vi "Panel Controller.vi"(5 "Show Event":refnum<user-event>, 7 "Stop Event":refnum<user-event>, 10 "Panel":refnum<class "Panel.lvclass">) -> ()   [LabVIEW 2017, in "1. Basic Panels.lvlib"]
doc: "This is a basic panel. \n\nIt doesn't know what type of panel it is until runtime, this means that whoever launches this VI can define what type of panel it will be.\n----\nCopyright: MGI 2016\nAuthor: Derek Trepanier"
uses:
  1. Basic Panels.lvlib
  panel-manager/Source/Panel/Panel.lvclass
  panel-manager/Source/Panel Helper/Panel Helper.lvclass
  panel-manager/Source/Deferer/Deferer.lvclass
  panel-manager/Source/Cursor/Cursor.lvclass
panel:
  out "Numeric":i32
  in  "Mouse Busy for 1000ms":bool
  in  "Mouse Busy for 500ms":bool
  in  "Defer for 1000ms":bool
  in  "Defer for 500ms":bool
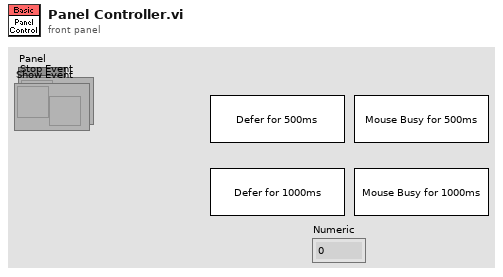
[diagram p1: front panel]
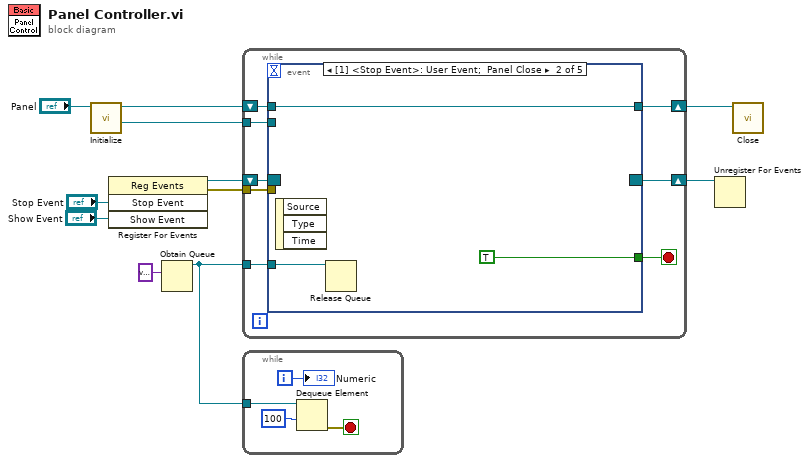
[diagram p0: block diagram]
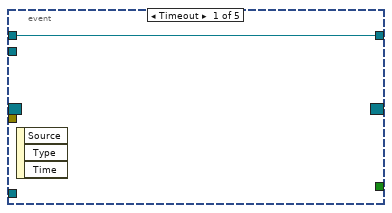
[diagram p2: hidden frame]
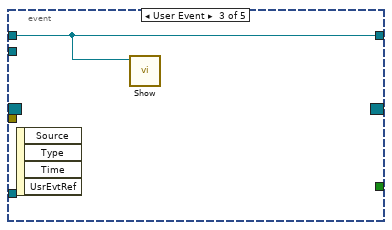
[diagram p3: hidden frame]
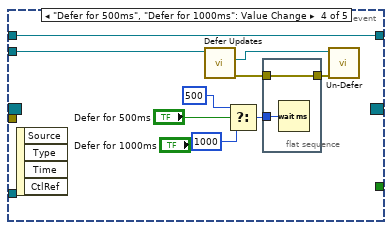
[diagram p4: hidden frame]
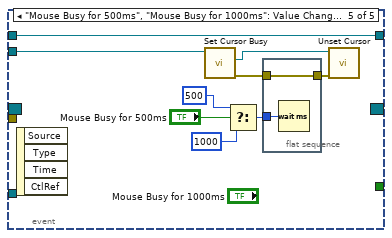
[diagram p5: hidden frame]
diagram:
  n1 = call "Initialize.vi"("Panel In"="Panel") -> ("My Helper out"=w3:refnum<class "Panel Helper.lvclass">, "Panel Out"=w8:refnum<class "Panel.lvclass">)  [unwired: 8 in, 1 out]
  n2 = register-events("Stop Event", "Show Event") -> (reference out=w9:refnum<event-registration>, error out=w4:errorcluster)  [unwired: 2 in]
  n3 = Obtain Queue(element data type=variant) -> (queue out=w1:refnum<queue>)  [unwired: 4 in, 2 out]
  n4 = while {
    tunnel: w4 -> [w15]
    shift-right: [w16] -> w6
    shift-left: w9 -> [w19]
    shift-right: [w17] -> w7
    shift-left: w8 -> [w18]
    tunnel: w3 -> [w13]
    tunnel: w1 -> [w12]
    stop <- w14 stop-if-true
    n5 = event shown="[1] <Stop Event>: User Event;  Panel Close" {
      selector: w19 -> [_ _ _ _ _]
      dyn-events: [_ _ _ _ _] -> w16
      timeout: _ -> [_ _ _ _ _]
      tunnel: w18 -> [w20 w23 w24 w33 w44]
      tunnel: [w20 w23 w24 w33 w44] -> w17
      tunnel: w15 -> [_ _ _ _ _]
      tunnel: [_ TRUE _ _ _] -> w14
      tunnel: w13 -> [_ _ _ w32 w43]
      tunnel: w12 -> [_ w21 _ _ _]
      event Timeout {
        n6 = event-data() -> ()  [unwired: 1 in, 3 out]
      }
      event User Event; Panel Close {
        n7 = event-data() -> ()  [unwired: 1 in, 3 out]
        n8 = Release Queue(queue=w21) -> ()  [unwired: 2 in, 3 out]
      }
      event User Event {
        n9 = event-data() -> ()  [unwired: 1 in, 4 out]
        n10 = call "Show.vi"("Panel in"=w24) -> ()  [unwired: 10 in, 1 out]
      }
      event "Defer for 500ms", "Defer for 1000ms": Value Change {
        n11 = event-data() -> ()  [unwired: 1 in, 4 out]
        n12 = call "Defer Updates.vi"("Controller in"=w32) -> ("Error Out"=w27:errorcluster, "Deferer"=w28:refnum<class "Deferer.lvclass">)  [unwired: 9 in]
        n13 = Select(t=u32 500 ("ms"), s="Defer for 500ms", f=u32 1000 ("ms")) -> (s? t:f=w25:u32)
        n14 = flat-sequence {
          tunnel: w25 -> [w35]
          tunnel: [w34] -> w26
          tunnel: w27 -> [w34]
          frame #0 {
            n15 = Wait (ms)(milliseconds to wait=w35) -> ()  [unwired: 1 out]
          }
        }
        n16 = call "Un-Defer.vi"("Error In"=w26, "Deferer in"=w28) -> ()  [unwired: 9 in, 1 out]
      }
      event "Mouse Busy for 500ms", "Mouse Busy for 1000ms": Value Change {
        n17 = event-data() -> ()  [unwired: 1 in, 4 out]
        n18 = call "Set Cursor Busy.vi"("Panel Helper in"=w43) -> ("error out"=w36:errorcluster, "Cursor"=w39:refnum<class "Cursor.lvclass">)  [unwired: 9 in]
        n19 = Select(t=u32 500 ("ms"), s="Mouse Busy for 500ms", f=u32 1000 ("ms")) -> (s? t:f=w38:u32)
        n20 = flat-sequence {
          tunnel: w38 -> [w46]
          tunnel: [w45] -> w37
          tunnel: w36 -> [w45]
          frame #0 {
            n21 = Wait (ms)(milliseconds to wait=w46) -> ()  [unwired: 1 out]
          }
        }
        n22 = call "Unset Cursor.vi"("error in (no error)"=w37, "Cursor in"=w39) -> ()  [unwired: 9 in, 1 out]
      }
    }
  }
  n23 = while {
    tunnel: w1 -> [w49]
    i -> [w50]
    stop <- w47 stop-if-true
    n24 = Dequeue Element(queue=w49, timeout in ms (-1)=100) -> (error out=w47:errorcluster)  [unwired: 1 in, 3 out]
    "Numeric" <- w50
  }
  n25 = Unregister For Events(event registration refnum=w6) -> ()  [unwired: 1 in, 1 out]
  n26 = call-dynamic "Close.vi"("Panel In"=w7) -> ()  [unwired: 10 in, 1 out]
